vi "Generate Weights.vi"(10 "Neurons":u32, 11 "Inputs":u32) -> (3 "Layer Weights":T1)   [LabVIEW 2011, in "Super Simple Neural Network.lvlib"]
uses:
  Super Simple Neural Network.lvlib
  Types/2D Array.ctl
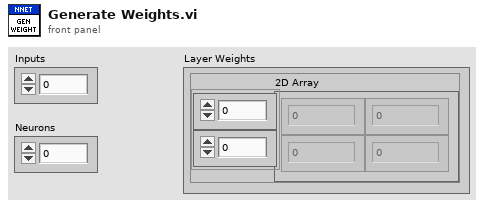
[diagram p1: front panel]
types:
  T1 = typedef "Super Simple Neural Network.lvlib/2D Array.ctl" = cluster{"2D Array":dbl[][]}
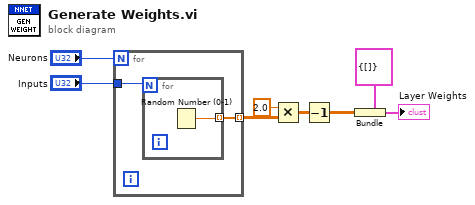
[diagram p0: block diagram]
diagram:
  n1 = for {
    N: "Neurons" -> [_]
    tunnel: [w10] -> w7 mode=indexing
    tunnel: "Inputs" -> [w9]
    n2 = for {
      N: w9 -> [_]
      tunnel: [w11] -> w10 mode=indexing
      n3 = Random Number (0-1)() -> (number: 0 to 1=w11:dbl)
    }
  }
  n4 = Multiply(x=2.0, y=w7) -> (x*y=w6:dbl[][])
  n5 = Decrement(x=w6) -> (x-1=w8:dbl[][])
  n6 = Bundle(cluster=T1 {"2D Array"=[]}, "2D Array"=w8) -> (→"Layer Weights":T1)
